vi "NISE.Write client handle.vi"(8 "error in (no error)":errorcluster, 10 "Client Handle":T1, 11 "SLSC Interface in":refnum<class "SLSC Interface.lvclass">) -> (0 "error out":errorcluster, 3 "SLSC Interface out":refnum<class "SLSC Interface.lvclass">)   [LabVIEW 2016, in "SLSC Interface.lvclass"]
uses:
  SLSC Interface.lvclass
  <vilib>/httpClient/ClientHandle.ctl
  SLSC Interface.lvclass/SLSC Interface.ctl
  <vilib>/httpClient/LabVIEWHTTPClient.lvlib
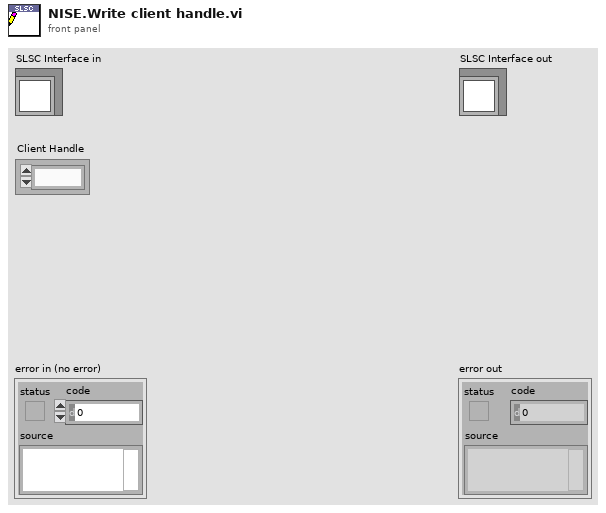
[diagram p1: front panel]
types:
  T1 = typedef "LabVIEWHTTPClient.lvlib/ClientHandle.ctl" = refnum<k1>
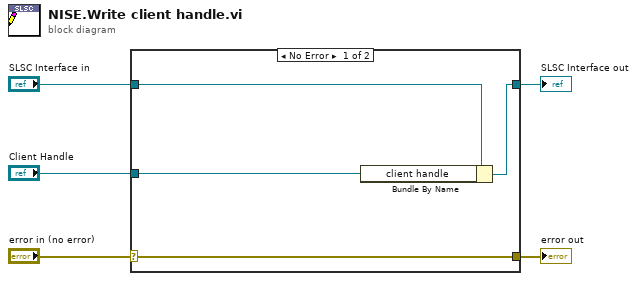
[diagram p0: block diagram]
diagram:
  n1 = case shown="No Error" "error in (no error)" {
    selector: "error in (no error)" -> [w9 w10]
    tunnel: [w9 w10] -> w4
    tunnel: [w7 w11] -> w2
    tunnel: "SLSC Interface in" -> [w8 w11]
    tunnel: "Client Handle" -> [w6 _]
    frame No Error {
      n2 = Bundle By Name(cluster=w8, "client handle"=w6) -> (w7:refnum<class "SLSC Interface.lvclass">)
    }
    frame Error {
    }
  }
  "error out" <- w4
  "SLSC Interface out" <- w2
